vi "Initialise RefDAQ Parameters.vi"(5 "AOL Global":T1={"Imaging Protocol"=enum."Live Imaging", "Number of POI"=0, "Number of Miniscans"=0, "Number of Trials"=0, "Number of Cycles "=0, "# Averaged Frames"=0, "Laser power (%)"=0, "Pockels (V)"=0.0, "Acquisition Length (sec)"=0.0, "Fill time (us)"=0.0, "POI Dwell time (us)"=0.0, "Miniscan Dwell time per pixel (us)"=0.0, "PMT 1"=0.0, "PMT 2"=0.0, "Back Apperture (mA)"=0.0, "Frame Size"=512, "Center Frequency"=0.0, "Field of View (um)"=175.0, "Field of View (norm)"=175.0, "DwellTime (us)"=0.0, "Ref Dwell Time (us)"=0.0, "Wavelength (nm)"=0.0, "Zoom"=1.0, "AOL Z"=0.0, "AOL Mode"=enum."Raster", "GridXY"=0.0, "GridZ"=0.0, "TriggerPeriod (sec)"=0.0, "Number of Pixels in Miniscan"=0, "Experiment folder path"=path "", "X centre"=0.0, "Y centre"=0.0, "Angle (degrees)"=0.0, "Angle Xs (degrees)"=0.0, "Angle Ys (degrees)"=0.0, "Plane Mode"=0, "Threshold"=[], "Regenerate Chirps"=FALSE, "Rectangle ROI length (pixels)"=0, "Rectangle ROI height (pixels)"=0, "AOD fill"=4900, "StartupDelay"=0, "Samples Wait after Trigger"=5080, "Slip Cycle"=600000, "Add Cycle"=TRUE, "Functional Mode"=enum."Point", "Z Start"=0.0, "Z Stop"=0.0, "# Planes"=0, "Total Pixels"=0, "Variable Miniscan Pixels"=[], "Use Variable Length"=FALSE, "Use Variable Resolution"=FALSE, "Laser power (%) at Z Start"=0, "Laser power (%) at Z Stop"=0, "Ref Z Step"=0} {"Angle Ys (degrees)" format="%#.6g"; "Angle Xs (degrees)" format="%#.6g"; "Plane Mode" items=["XY Plane", "XZ Plane", "YZ Plane", "arbitraryplane"]; "Frame Size" items=["100X100"=100, "128X128"=128, "200X200"=200, "256X256"=256, "512X512"=512, "1024x1024"=1024, "2048x2048"=2048]; "Back Apperture (mA)" format="%#.6g"; "Pockels (V)" format="%#.6g"; "PMT 2" format="%#.6g"; "PMT 1" format="%#.6g"; "Angle (degrees)" format="%#.6g"; "POI Dwell time (us)" format="%#.6g"}, 11 "error in (no error)":errorcluster) -> (4 "Refnum out":T7, 15 "error out":errorcluster)   [LabVIEW 2020]
uses:
  RIG-SPECIFIC FILES/FPGA Refs/FPGA Ref.ctl
  Typedefs/Controls/AOL_Globals.ctl
  Typedefs/Imaging Protocols enum.ctl
  Typedefs/Frame Size.ctl
  Typedefs/AOL modes.ctl
  Typedefs/Plane Mode.ctl
  Typedefs/Functional Mode.ctl
  Typedefs/HW config states enum.ctl
  Global Variables/General Globals.vi
  Peripherals Control/Pockels/Globals/gl_Pockels control globals.vi
  <vilib>/Utility/error.llb/Error Cluster From Error Code.vi
  <vilib>/rvi/errors/niLvFpgaAdjustHostInterfaceError.vi
  <vilib>/rvi/interface/nirviReadWriteControl/nirviReadWriteControl.xnode
  <vilib>/rvi/interface/nirviMethod/nirviMethod.xnode
  <vilib>/rvi/errors/niLvFpgaMergeErrorWithErrorCode.vi
  NiFpgaLv.dll
  <vilib>/rvi/interface/Simulation/niFpgaSimulationCallBeginRW.vi
  <vilib>/FPGAPlugInAG/Dynamic/niLvFpga_StopFifo_Dynamic.vi
  <vilib>/FPGAPlugInAG/Dynamic/niLvFpga_StartFifo_Dynamic.vi
panel:
  out "scan_int":fxp<+,16,2>
  out "mc_delay prog":u16=1525
  in  "diff_thresh_z":fxp<+/-,16,8>
  in  "use sliding average":bool
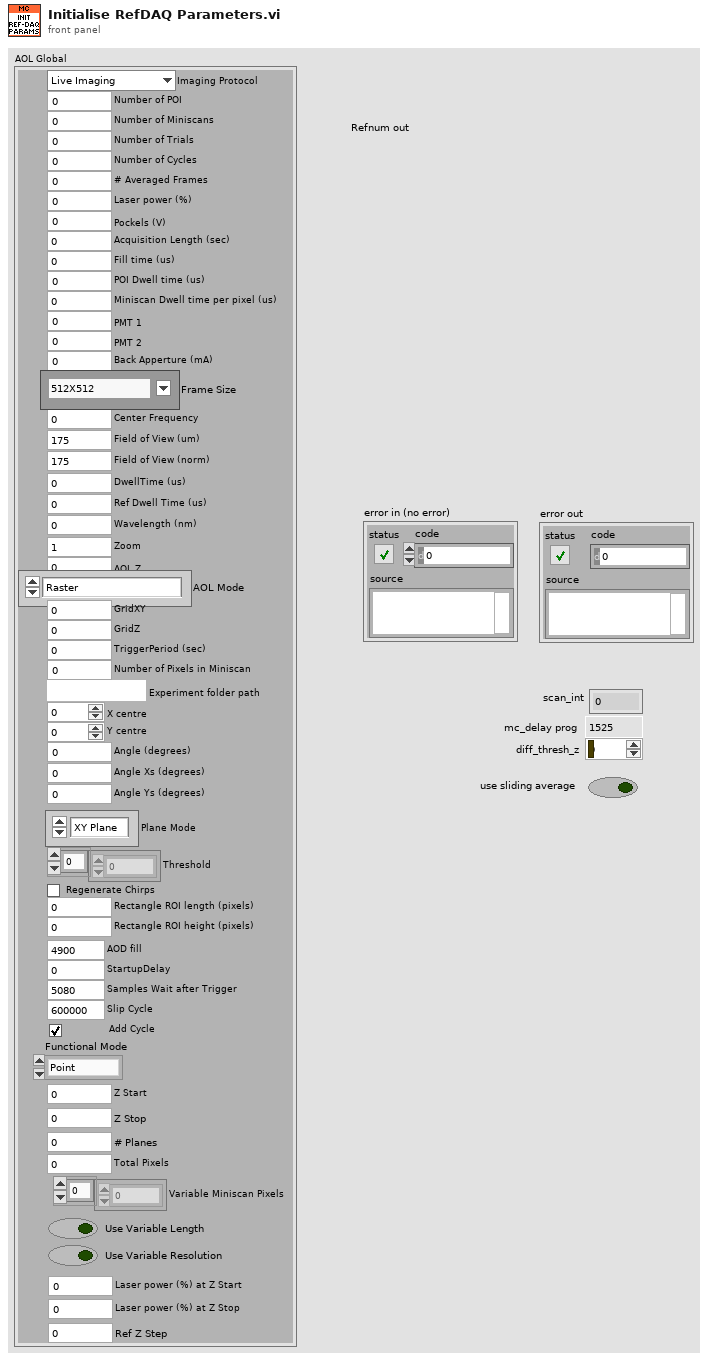
[diagram p1: front panel]
types:
  T1 = typedef "AOL_Globals.ctl" = cluster{"Imaging Protocol":T2, "Number of POI":u16, "Number of Miniscans":u16, "Number of Trials":u16, "Number of Cycles ":u64, "# Averaged Frames":u16, "Laser power (%)":u8, "Pockels (V)":dbl, "Acquisition Length (sec)":dbl, "Fill time (us)":dbl, "POI Dwell time (us)":dbl, "Miniscan Dwell time per pixel (us)":dbl, "PMT 1":dbl, "PMT 2":dbl, "Back Apperture (mA)":dbl, "Frame Size":T3, "Center Frequency":dbl, "Field of View (um)":dbl, "Field of View (norm)":dbl, "DwellTime (us)":dbl, "Ref Dwell Time (us)":dbl, "Wavelength (nm)":dbl, "Zoom":dbl, "AOL Z":dbl, "AOL Mode":T4, "GridXY":dbl, "GridZ":dbl, "TriggerPeriod (sec)":dbl, "Number of Pixels in Miniscan":u16, "Experiment folder path":path, "X centre":dbl, "Y centre":dbl, "Angle (degrees)":dbl, "Angle Xs (degrees)":dbl, "Angle Ys (degrees)":dbl, "Plane Mode":T5, "Threshold":u16[], "Regenerate Chirps":bool, "Rectangle ROI length (pixels)":u16, "Rectangle ROI height (pixels)":u16, "AOD fill":u16, "StartupDelay":i32, "Samples Wait after Trigger":u16, "Slip Cycle":u32, "Add Cycle":bool, "Functional Mode":T6, "Z Start":dbl, "Z Stop":dbl, "# Planes":i32, "Total Pixels":i32, "Variable Miniscan Pixels":u16[], "Use Variable Length":bool, "Use Variable Resolution":bool, "Laser power (%) at Z Start":u8, "Laser power (%) at Z Stop":u8, "Ref Z Step":i8}
  T2 = typedef "Imaging Protocols enum.ctl" = enum16{"AOL Z-Stack", "Motor Z Stack", "Parameter Sweep", "Functional Acquisition", "Single Plane Acquisition", "Volume Acquisition", "Live Imaging", "Live Plane Imaging", "Live Volume Imaging"}
  T3 = typedef "Frame Size.ctl" = u16
  T4 = typedef "AOL modes.ctl" = enum16{"Raster", "Structural", "Pointing", "Mini Scan", "Alignment"}
  T5 = typedef "Plane Mode.ctl" = u16
  T6 = typedef "Functional Mode.ctl" = enum16{"Point", "Line", "Patch", "Plane", "Volume"}
  T7 = typedef "FPGA Ref.ctl" = refnum<k20>
  T8 = typedef "HW config states enum.ctl" = enum16{"Load from file", "Save to file", "Save backup", "Write all", "Read all", "Write XY stage settings", "Write DAQ FPGA settings", "Write Control FPGA settings", "Write Phys Channels", "Write System Config", "Write HW Config", "Save System Config", "Save HW Config", "Clear", "Compare from file"}
  T9 = typedef "Hardware Configuration settings.ctl" = cluster{"Dev. PC":bool, "Swap XY on stage":bool, "No of AOD":u8, "MC Supported":bool, "Axial MC":bool, "Computer MAC address":string, "Externalise Triggers":bool, "Trigger HW config":T10, "DAQmx Chan":T11, "XYZ Stage Control Config":T12, "XY stage available":bool, "XY Comms Config Cluster":T13, "Y stage available":bool, "Y Comms Config Cluster":T13, "Z stage available":bool, "Z Comms Config Cluster ":T13, "Encoder available":bool, "Encoder":T15, "VidRec available":bool, "Cam VidRec":T16, "Laser Power Control HW config":T17, "Laser 1 available":bool, "Laser 1 config cluster":T18, "Prechirper 1 available":bool, "Prechirper 1 config cluster":T19, "Control system.FPGA available?":bool, "Control Sys. HW config":T20, "DAQ FPGA HW Config":T21, "PMT Control Voltage Limits":T24}
  T10 = typedef "Triggers HW config.ctl" = cluster{"Available Device List":i32, "Device Address":string}
  T11 = typedef "DAQmx physical channels cluster.ctl" = cluster{"Pockels AO":tag, "Hard shutter AO":tag, "PMT AOs":tag, "Galvo AOs":tag, "Power meter AI":tag}
  T12 = typedef "XYZControlConfig.ctl" = enum16{"None", "XYZ", "XY-Z", "X-Y-Z", "Z"}
  T13 = typedef "Peripherals comms config cluster.ctl" = cluster{"Name":string, "Device Address":string, "Port ":u16, "Baudrate":i32, "Comms Type":T14}
  T14 = typedef "Comms Type.ctl" = enum16{"GPIB-IEEE488", "Serial-RS232", "Serial-RS485", "Serial-RS422", "Serial-USB", "Ethernet-TCP/IP", "Ethernet-UDP"}
  T15 = typedef "Encoder config cluster.ctl" = cluster{"IP address":string, "Port":u16, "Wheel radius (cm)":dbl, "Encoder Trigger":tag}
  T16 = typedef "Cam VidRec HW config setup cluster.ctl" = cluster{"DO flag-Video record":tag, "DO flag-Trial start":tag}
  T17 = typedef "Laser Power Control HW config.ctl" = cluster{"Laser Power Control":string, "Laser Power Modulation Control":enum16{"NI", "FPGA"}}
  T18 = typedef "Laser 1 config cluster.ctl" = cluster{"COM port":refnum<visa-resource-name>, "Baud Rate":i32, "Type":string}
  T19 = typedef "PreChirper 1 config cluster.ctl" = cluster{"Type":string, "Baud Rate":i32, "COM port":refnum<visa-resource-name>}
  T20 = typedef "Control Sys HW config cluster.ctl" = cluster{"Control system.FPGA Type":enum16{"Virtex 5", "Virtex 7"}, "Control system.Network adapter name":string, "Control system.MAC address":string, "Control system.Ethernet Port":u32, "Control system.Ethernet Port Opened":bool}
  T21 = typedef "DAQ FPGA HW config cluster.ctl" = cluster{"FGPA Ref":T7, "Target":T22, "input card type":T23}
  T22 = typedef "nirio_resource_hc.ctl" = tag
  T23 = typedef "FPGA input type AC-DC.ctl" = enum16{"AC Card", "DC Card"}
  T24 = typedef "PMT Control Voltage limits.ctl" = cluster{"Lower Limit":dbl, "Upper Limit":dbl}
  T25 = typedef "Ref DAQ Param.ctl" = cluster{"Full Frame Size":u16, "Ref Field of View":sgl, "Ref Zoom":i8, "Ref_dwellTime":sgl, "Ref X-pixels-per-line(Npxr)":i16, "Ref Y-lines-per-image(Npyr)":i16, "Ref Z-lines-per-image":i16, "Ignore Z lines":i16, "Ref Scan Cycles":i32, "Ref threshold XY":u16, "Ref threshold Z":u16, "Ref average XY":u16, "Ref Average  Z":u16, "Proportional_scale":fxp<+,16,2>, "Integral_scale":fxp<+/-,16,12>, "Proportional_scale Z":fxp<+,16,2>, "Integral_scale Z":fxp<+/-,16,12>, "Diff_threshold":fxp<+,16,2>, "Diff_threshold _z":fxp<+,16,2>, "Sliding Average":bool, "Ref count reset enabled":bool, "Auto-centering":bool}
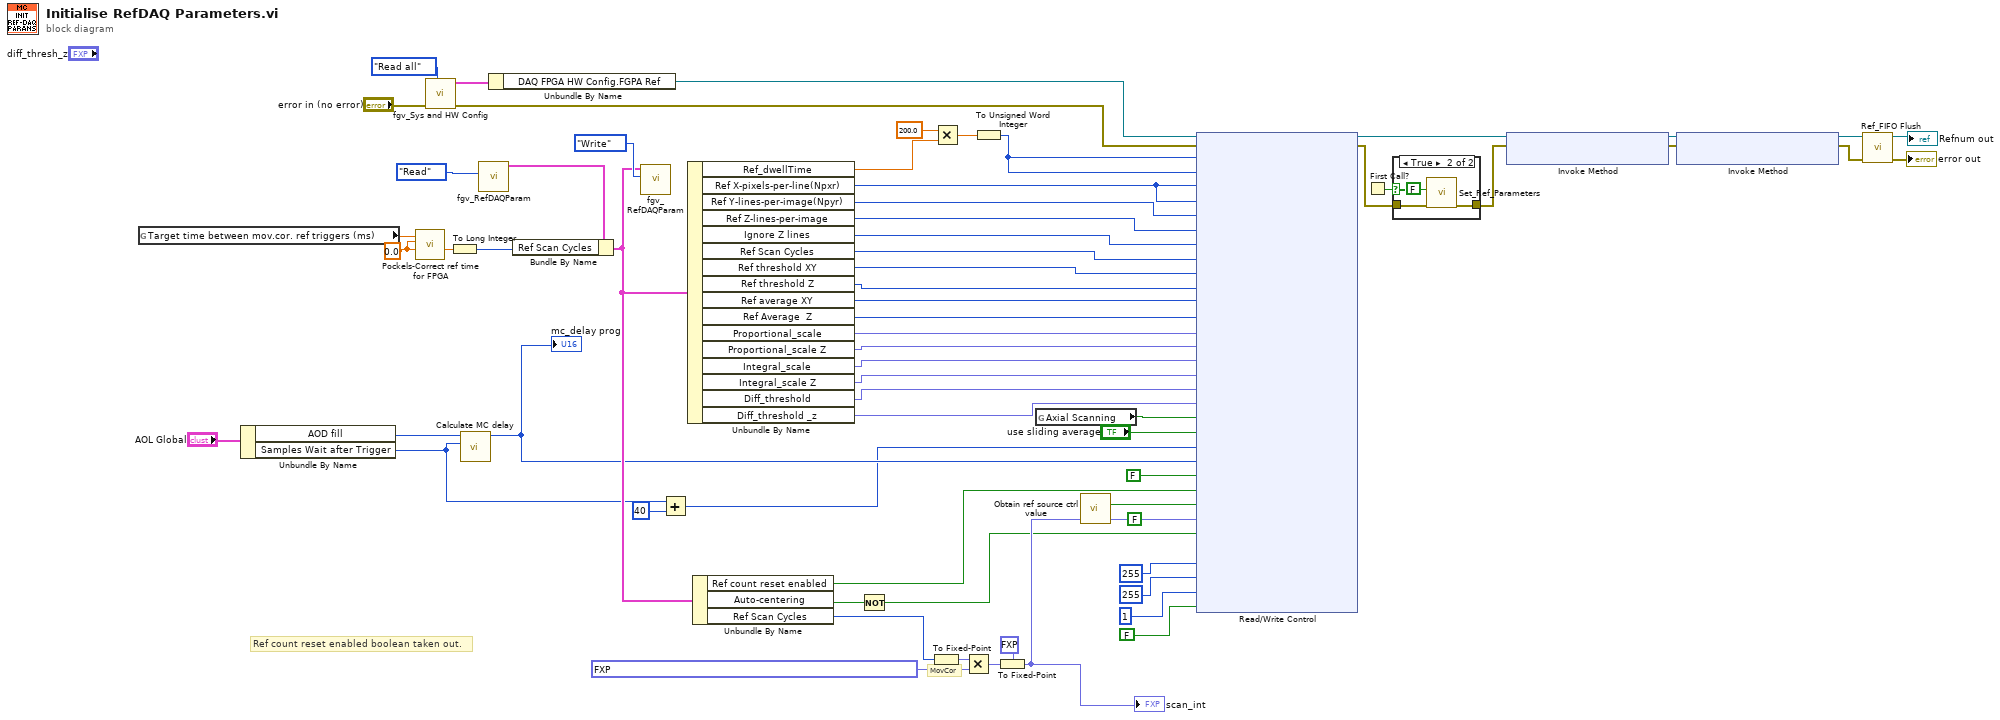
[diagram p0: block diagram]
diagram:
  w22 = 0.0 ("Time for main img line OR for a single POI (ms)")
  # "Ref count reset enabled boolean taken out."
  # "MovCor"
  n1 = global read "gl_Pockels control globals.vi" "Target time between mov.cor. ref triggers (ms)"() -> (w24:dbl)
  n2 = Unbundle By Name("AOL Global") -> ("AOD fill"=w32:u16, "Samples Wait after Trigger"=w6:u16)
  n3 = call "Pockels-Correct ref time for FPGA.vi"("Fine tuning multiplier"=w22, "Time for main img line OR for a single POI (ms)"=w22, "Actual resulting time between ref triggers (ms)"=w24) -> ("Ref Scan Cycles"=w23:dbl)  [unwired: 7 in, 1 out]
  n4 = call "fgv_Sys and HW Config.vi"("Function"=HW_config_states_enum."Read all", "error in (no error)"="error in (no error)") -> ("error out"=w42:errorcluster, "Hardware Configuration OUT"=w44:T9)  [unwired: 7 in, 1 out]
  n5 = To Long Integer(number=w23) -> (32bit integer=w21:i32)
  n6 = call "Calculate MC delay.vi"("Cycles to wait after trigger"=w6, "AOD Fill"=w32) -> ("mc delay prog read"=w31:u16)  [unwired: 9 in]
  "mc_delay prog" <- w31
  n7 = call "fgv_RefDAQParam.vi"("Function"=enum16{"Initialize", "Write", "Read"}."Read" ("Status")) -> ("RefDAQParam"=w57:T25)  [unwired: 9 in, 1 out]
  n8 = Unbundle By Name(w44) -> ("DAQ FPGA HW Config.FGPA Ref"=w43:T7)
  n9 = Bundle By Name(cluster=w57, "Ref Scan Cycles"=w21) -> (w54:T25)
  n10 = call "fgv_RefDAQParam.vi"("Function"=enum16{"Initialize", "Write", "Read"}."Write" ("Status"), "RefDAQParam in"=w54) -> ()  [unwired: 8 in, 2 out]
  n11 = Add(x=w6, y=u16 40) -> (x+y=w4:u16)
  n12 = Unbundle By Name(w54) -> ("Ref_dwellTime"=w64:sgl, "Ref X-pixels-per-line(Npxr)"=w14:i16, "Ref Y-lines-per-image(Npyr)"=w12:i16, "Ref Z-lines-per-image"=w11:i16, "Ignore Z lines"=w8:i16, "Ref Scan Cycles"=w13:i32, "Ref threshold XY"=w25:u16, "Ref threshold Z"=w20:u16, "Ref average XY"=w10:u16, "Ref Average  Z"=w9:u16, "Proportional_scale"=w19:fxp<+,16,2>, "Proportional_scale Z"=w18:fxp<+,16,2>, "Integral_scale"=w17:fxp<+/-,16,12>, "Integral_scale Z"=w16:fxp<+/-,16,12>, "Diff_threshold"=w56:fxp<+,16,2>, "Diff_threshold _z"=w55:fxp<+,16,2>)
  n13 = Unbundle By Name(w54) -> ("Ref count reset enabled"=w7:bool, "Auto-centering"=w2:bool, "Ref Scan Cycles"=w3:i32)
  n14 = Not(x=w2) -> (.not. x?=w1:bool)
  n15 = To Fixed-Point(number=w3) -> (fixed-point=w50:fxp<+/-,32,32>)  [unwired: 1 in]
  n16 = Multiply(x=sgl 200.0, y=w64) -> (x*y=w65:sgl)
  n17 = Multiply(x=w50, y=fxp<+,64,2> 4.999999999970306e-09 ("fixed-point type")) -> (x*y=w51:fxp<+/-,64,35>)
  n18 = To Unsigned Word Integer(number=w65) -> (unsigned 16bit integer=w15:u16)
  n19 = To Fixed-Point(fixed-point type=fxp<+,16,2> 0.0, number=w51) -> (fixed-point=w48:fxp<+,16,2>)
  "scan_int" <- w48
  n20 = global read "General Globals.vi" "Axial Scanning"() -> (w59:bool)
  n21 = call "Obtain ref source ctrl value.vi"() -> ("select_ref_red"=w53:bool)  [unwired: 11 in]
  n22 = xnode ("Read/Write Control")("FPGA VI Reference In"=w43, "error in"=w42, "Ref samps-per-pix (Pr)"=w15, "Ref samps-per-pix_z"=w15, "Ref x-pixels-per-line (Npxr)"=w14, "ref_z_pixels_per_line"=w14, "Ref y-pixels-per-line (Npyr)"=w12, "Ref _z_lines"=w11, "ignore_z_lines"=w8, "Ref Scan Cycles"=w13, "threshold_xy"=w25, "threshold_z"=w20, "Average"=w10, "Average Z"=w9, "proportioanl_scale"=w19, "proportioanl_scale _z"=w18, "Integral_scale_ind"=w17, "Integral_scale z"=w16, "diff_thresh"=w56, "diff_thresh_z"=w55, "Enable_ZMC"=w59, "use sliding average"="use sliding average", "samples wait after pulse"=w4, "mc_delay prog"=w31, "stop_background"=FALSE ("stop bg MC"), "Ref count reset enabled"=w7, "select_ref_red"=w53, "scan_int"=w48, "capture_ref_z"=w1, "enable_mc_recovery"=FALSE, "ref_diff_z"=u8 255, "ref_diff_x_y"=u8 255, "Average  offsets"=u16 1, "use_vel_estimate"=FALSE) -> ("FPGA VI Reference Out"=w33:T7, "error out"=w46:errorcluster)
  n23 = First Call?() -> (First Call?: T/F=w47:bool)
  n24 = case shown="True" w47 {
    tunnel: w46 -> [w67 w69]
    tunnel: [w67 w68] -> w34
    frame False {
    }
    frame True {
      n25 = call "Set_Ref_Parameters.vi"("error in"=w69, "use_increment_halfrate"=FALSE) -> ("error out"=w68:errorcluster)  [unwired: 7 in, 2 out]
    }
  }
  n26 = xnode ("Invoke Method")("FPGA VI Reference In"=w33, "error in"=w34) -> ("FPGA VI Reference Out"=w36:T7, "error out"=w35:errorcluster)
  n27 = xnode ("Invoke Method")("FPGA VI Reference In"=w36, "error in"=w35) -> ("FPGA VI Reference Out"=w39:T7, "error out"=w40:errorcluster)
  n28 = call "Ref_FIFO Flush.vi"("Error In"=w40, "FPGA VI Ref"=w39) -> ("Error Out"=→"error out":errorcluster, "FPGA VI Reference Out"=→"Refnum out":T7)  [unwired: 8 in]
